vi "Evaluate Part 1.vi"() -> ()   [LabVIEW 2021]
uses:
  Proto/Proto.lvclass
panel:
  out "Area":u64
  in  "Input":string
  # "2738 too low"
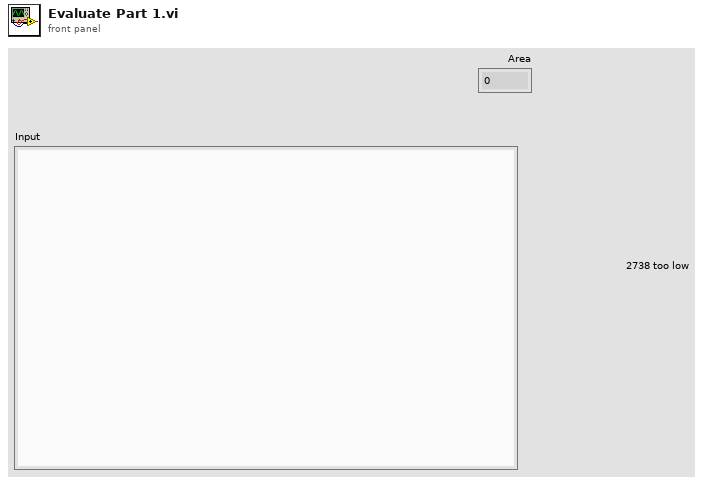
[diagram p1: front panel]
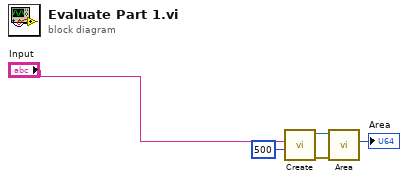
[diagram p0: block diagram]
diagram:
  n1 = call "Create.vi"("offset"=500, "Input"="Input") -> ("error out"=w4:errorcluster, "Proto"=w5:refnum<class "Proto.lvclass">)  [unwired: 8 in]
  n2 = call "Area.vi"("error in (no error)"=w4, "Proto in"=w5) -> ("Area"=→"Area":u64)  [unwired: 7 in, 2 out]
